vi "MessageName.vi"() -> (2 "MessageName":string)   [LabVIEW 2020, in "RequestTwoDouble.lvlib"]
uses:
  RequestTwoDouble.lvlib
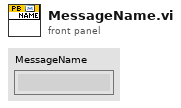
[diagram p1: front panel]
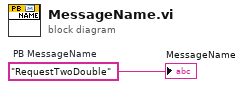
[diagram p0: block diagram]
diagram:
  w1 = "RequestTwoDouble"  # PB MessageName
  "MessageName" <- w1
